vi "Read Banner Text.vi"(8 "error in (no error)":errorcluster, 11 "New QControl Info in":refnum<class "New QControl Info.lvclass">) -> (0 "error out":errorcluster, 2 "Banner Text":string, 3 "New QControl Info out":refnum<class "New QControl Info.lvclass">)   [LabVIEW 2020, in "New QControl Info.lvclass"]
uses:
  New QControl Info.lvclass
  New QControl Info.lvclass/New QControl Info.ctl
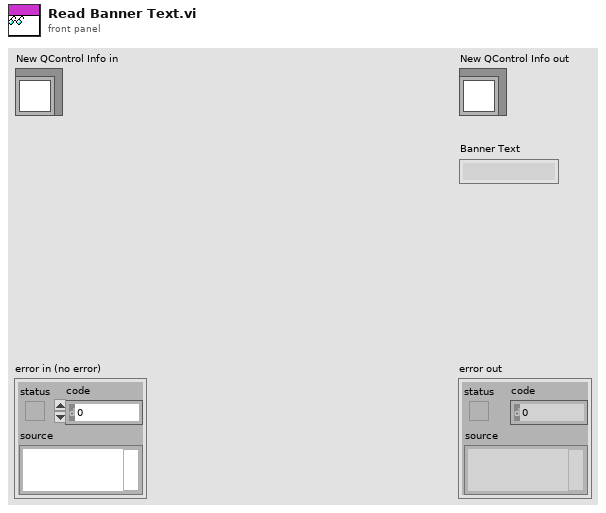
[diagram p1: front panel]
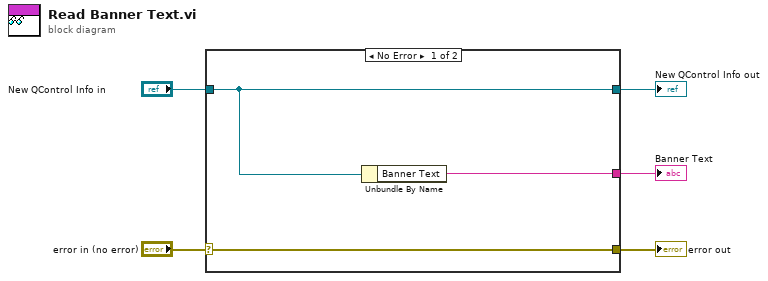
[diagram p0: block diagram]
diagram:
  n1 = case shown="No Error" "error in (no error)" {
    selector: "error in (no error)" -> [w8 w9]
    tunnel: [w8 w9] -> w4
    tunnel: [w7 w10] -> w2
    tunnel: "New QControl Info in" -> [w7 w10]
    tunnel: [w6 _] -> w1
    frame No Error {
      n2 = Unbundle By Name(w7) -> ("Banner Text"=w6:string)
    }
    frame Error {
    }
  }
  "error out" <- w4
  "New QControl Info out" <- w2
  "Banner Text" <- w1
